vi "Loop_SM.vi"() -> ()   [LabVIEW 2017, in "TemplateActuator.lvlib"]
uses:
  TemplateActuator.lvlib
  Globals/Global_STOP.vi
  ENUM_Action.ctl
  ENUM_State.ctl
  Cluster_CMD to SM Data.ctl
  Cluster_HW Status.ctl
  Global_CMD Data.vi
  Global_HW_Data Out.vi
  Cluster_SM To HW Data.ctl
  Cluster_SM Status.ctl
  Global_SM_Data Out.vi
  ENUM_SM Cmd Select.ctl
panel:
  out "SM Status_OUT":T1
  out "HW Data_OUT":T2
  out "Action":T3
  out "HW_Status":T4
  out "CMD_SM":T5
  out "Current State":T7
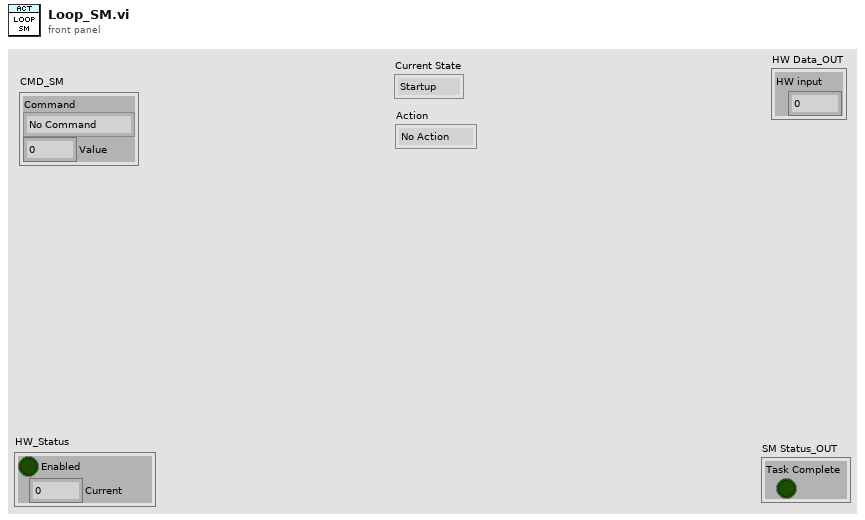
[diagram p1: front panel]
types:
  T1 = typedef "TemplateActuator.lvlib/Cluster_SM Status.ctl" = cluster{"Task Complete":bool}
  T2 = typedef "TemplateActuator.lvlib/Cluster_SM To HW Data.ctl" = cluster{"HW input":dbl}
  T3 = typedef "TemplateActuator.lvlib/ENUM_Action.ctl" = enum16{"No Action", "Reset Time", "Reset All", "Stop Action", "Set Action"}
  T4 = typedef "TemplateActuator.lvlib/Cluster_HW Status.ctl" = cluster{"Enabled":bool, "Current":dbl}
  T5 = typedef "TemplateActuator.lvlib/Cluster_CMD to SM Data.ctl" = cluster{"Command":T6, "Value":dbl}
  T6 = typedef "TemplateActuator.lvlib/ENUM_SM Cmd Select.ctl" = enum16{"No Command", "Stop", "Go"}
  T7 = typedef "TemplateActuator.lvlib/ENUM_State.ctl" = enum16{"Startup", "Idle", "Run", "Shutdown"}
  T8 = cluster{"Actions":T3[], "State":T7, "Current Time":timestamp, "Start Time":timestamp, "Loop Time (ms)":u32, "CMD_SM":T5, "HW_Status":T4, "HW Data_OUT":T2, "SM Status_OUT":T1}
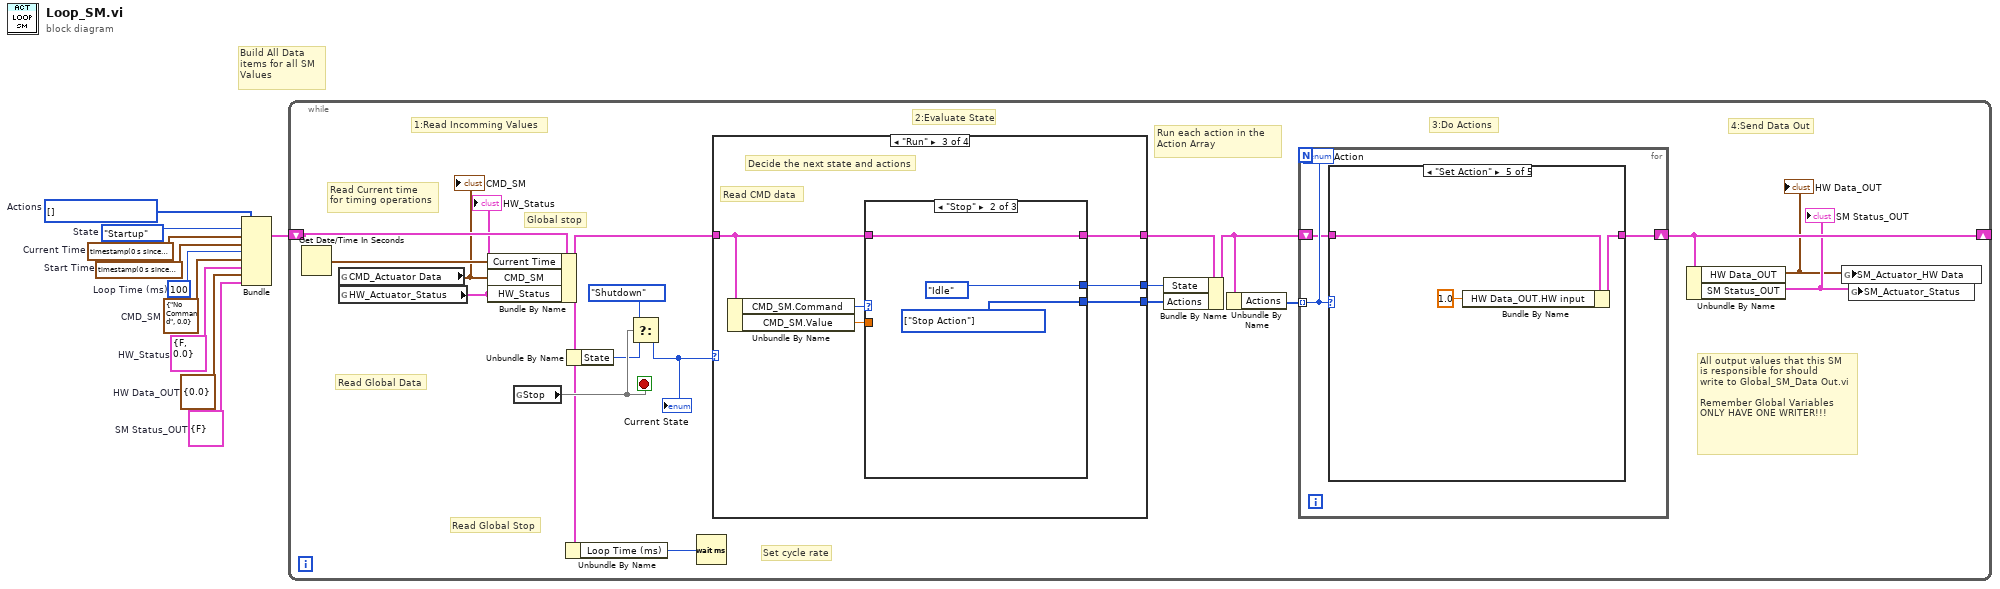
[diagram p0: block diagram]
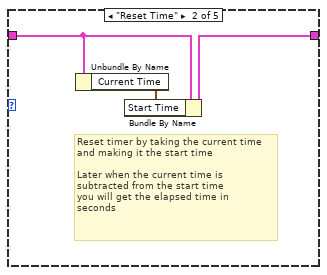
[diagram p3: hidden frame]
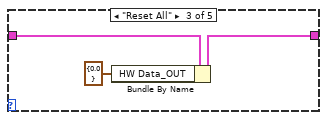
[diagram p4: hidden frame]
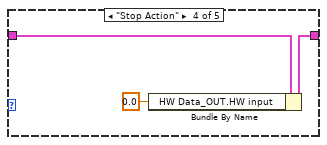
[diagram p5: hidden frame]
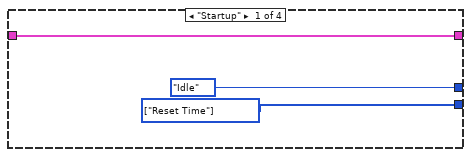
[diagram p6: hidden frame]
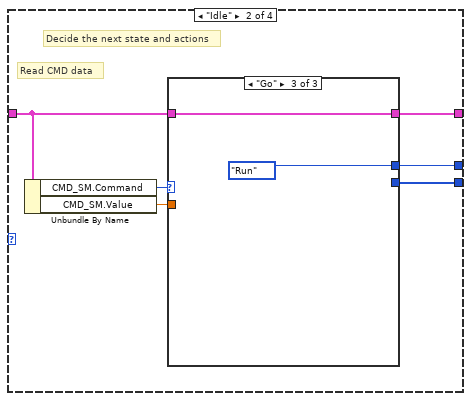
[diagram p7: hidden frame]
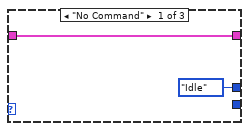
[diagram p8: hidden frame]
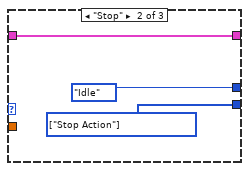
[diagram p9: hidden frame]
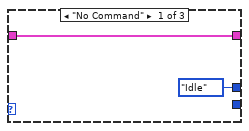
[diagram p10: hidden frame]
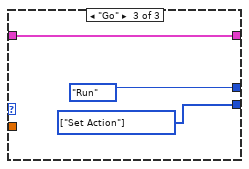
[diagram p11: hidden frame]
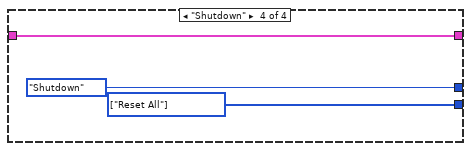
[diagram p12: hidden frame]
diagram:
  w1 = T1 {"Task Complete"=FALSE}  # SM Status_OUT
  w2 = T2 {"HW input"=0.0}  # HW Data_OUT
  w3 = T4 {"Enabled"=FALSE, "Current"=0.0}  # HW_Status
  w4 = T5 {"Command"=enum."No Command", "Value"=0.0}  # CMD_SM
  w5 = u32 100  # Loop Time (ms)
  w6 = T3[] [] items=["No Action", "Reset Time", "Reset All", "Stop Action", "Set Action"]  # Actions
  w7 = timestamp(0 s since 1904-01-01)  # Start Time
  w8 = timestamp(0 s since 1904-01-01)  # Current Time
  w9 = ENUM_State."Startup"  # State
  # "Build All Data items for all SM Values"
  n1 = Bundle("Actions"=w6, "State"=w9, "Current Time"=w8, "Start Time"=w7, "Loop Time (ms)"=w5, "CMD_SM"=w4, "HW_Status"=w3, "HW Data_OUT"=w2, "SM Status_OUT"=w1) -> (w10:T8)  [unwired: 1 in]
  n2 = while {
    shift-right: [w17] -> _
    shift-left: w10 -> [w27]
    stop <- w21 stop-if-true
    # "Read Global Data"
    # "Set cycle rate"
    # "All output values that this SM\nis responsible for should\nwrite to Global_SM_Data Out.vi\n\nRemember Global Variables\nONLY HAVE ONE WRITER!!!"
    # "Read Current time\nfor timing operations"
    # "Run each action in the Action Array"
    # "Read Global Stop"
    # "1:Read Incomming Values"
    # "2:Evaluate State"
    # "3:Do Actions"
    # "4:Send Data Out"
    # "Global stop"
    n3 = Get Date/Time In Seconds() -> (seconds since 1Jan1904=w26:timestamp)
    n4 = global read "Global_CMD Data.vi" "CMD_Actuator Data"() -> (w14:T5)
    "CMD_SM" <- w14
    n5 = global read "Global_HW_Data Out.vi" "HW_Actuator_Status"() -> (w13:T4)
    "HW_Status" <- w13
    n6 = Bundle By Name(cluster=w27, "Current Time"=w26, "CMD_SM"=w14, "HW_Status"=w13) -> (w15:T8)
    n7 = global read "Global_Stop.vi" "Stop"() -> (w21)
    n8 = Unbundle By Name(w15) -> ("Loop Time (ms)"=w16:u32)
    n9 = Unbundle By Name(w15) -> ("State"=w19:T7)
    n10 = Select(t=ENUM_State."Shutdown" ("State"), s=w21, f=w19) -> (s? t:f=w18:T7)
    "Current State" <- w18
    n11 = Wait (ms)(milliseconds to wait=w16) -> ()  [unwired: 1 out]
    n12 = case shown="\"Run\"" w18 {
      tunnel: w15 -> [w47 w52 w65 w77]
      tunnel: [w47 w51 w64 w77] -> w24
      tunnel: [ENUM_State."Idle" ("State") w49 w62 ENUM_State."Shutdown" ("State")] -> w23
      tunnel: [w46 w48 w61 w75] -> w22
      frame "Startup" {
        w46 = T3[] [enum."Reset Time"] items=["No Action", "Reset Time", "Reset All", "Stop Action", "Set Action"] ("Actions")
      }
      frame "Idle" {
        # "Read CMD data"
        # "Decide the next state and actions"
        n13 = Unbundle By Name(w52) -> ("CMD_SM.Command"=w53:T6, "CMD_SM.Value"=w50:dbl)
        n14 = case shown="\"Go\"" w53 {
          tunnel: w52 -> [w55 w58 w60]
          tunnel: [w55 w58 w60] -> w51
          tunnel: w50 -> [_ _ _]
          tunnel: [ENUM_State."Idle" ("State") ENUM_State."Idle" ("State") ENUM_State."Run" ("State")] -> w49
          tunnel: [_ w56 _] -> w48
          frame "No Command" {
          }
          frame "Stop" {
            w56 = T3[] [enum."Stop Action"] items=["No Action", "Reset Time", "Reset All", "Stop Action", "Set Action"] ("Actions")
          }
          frame "Go" {
          }
        }
      }
      frame "Run" {
        # "Read CMD data"
        # "Decide the next state and actions"
        n15 = Unbundle By Name(w65) -> ("CMD_SM.Command"=w66:T6, "CMD_SM.Value"=w63:dbl)
        n16 = case shown="\"Stop\"" w66 {
          tunnel: w65 -> [w68 w71 w74]
          tunnel: [w68 w71 w74] -> w64
          tunnel: w63 -> [_ _ _]
          tunnel: [ENUM_State."Idle" ("State") ENUM_State."Idle" ("State") ENUM_State."Run" ("State")] -> w62
          tunnel: [_ w69 w72] -> w61
          frame "No Command" {
          }
          frame "Stop" {
            w69 = T3[] [enum."Stop Action"] items=["No Action", "Reset Time", "Reset All", "Stop Action", "Set Action"] ("Actions")
          }
          frame "Go" {
            w72 = T3[] [enum."Set Action"] items=["No Action", "Reset Time", "Reset All", "Stop Action", "Set Action"] ("Actions")
          }
        }
      }
      frame "Shutdown" {
        w75 = T3[] [enum."Reset All"] items=["No Action", "Reset Time", "Reset All", "Stop Action", "Set Action"] ("Actions")
      }
    }
    n17 = Bundle By Name(cluster=w24, "State"=w23, "Actions"=w22) -> (w25:T8)
    n18 = Unbundle By Name(w25) -> ("Actions"=w28:T3[])
    n19 = for {
      tunnel: w28 -> [w31] mode=indexing
      shift-right: [w30] -> w17
      shift-left: w25 -> [w29]
      n20 = case shown="\"Set Action\"" w31 {
        tunnel: w29 -> [w32 w35 w38 w41 w44]
        tunnel: [w32 w34 w37 w40 w43] -> w30
        frame "No Action" {
        }
        frame "Reset Time" {
          # "Reset timer by taking the current time\nand making it the start time\n\nLater when the current time is \nsubtracted from the start time\nyou will get the elapsed time in \nseconds"
          n21 = Unbundle By Name(w35) -> ("Current Time"=w33:timestamp)
          n22 = Bundle By Name(cluster=w35, "Start Time"=w33) -> (w34:T8)
        }
        frame "Reset All" {
          n23 = Bundle By Name(cluster=w38, "HW Data_OUT"=T2 {"HW input"=0.0}) -> (w37:T8)
        }
        frame "Stop Action" {
          n24 = Bundle By Name(cluster=w41, "HW Data_OUT.HW input"=0.0) -> (w40:T8)
        }
        frame "Set Action" {
          n25 = Bundle By Name(cluster=w44, "HW Data_OUT.HW input"=1.0) -> (w43:T8)
        }
      }
      "Action" <- w31
    }
    n26 = Unbundle By Name(w17) -> ("HW Data_OUT"=w11:T2, "SM Status_OUT"=w12:T1)
    "HW Data_OUT" <- w11
    "SM Status_OUT" <- w12
    n27 = global write "Global_SM_Data Out.vi" "SM_Actuator_HW Data"(w11) -> ()
    n28 = global write "Global_SM_Data Out.vi" "SM_Actuator_Status"(w12) -> ()
  }
